vi "Sensor_Reads.vi"() -> ()   [LabVIEW 2020]
uses:
  <vilib>/Rock Robotics/WPI/ThirdParty/Phoenix-LabVIEW/Pigeon IMU/CTRE_PigeonIMU_TareType.ctl
  <vilib>/Rock Robotics/Network Tables/NT Read Number.vi
  Globals/Sensor_Values.vi
  Hardware/Drive/Drive_Hardware_Globals.vi
  Globals/Drive_Globals.vi
  <vilib>/Rock Robotics/Network Tables/NT Write Number.vi
  <vilib>/Rock Robotics/WPI/ThirdParty/Phoenix-LabVIEW/Pigeon IMU/CTRE_PigeonIMU_GetYPR.vi
  <vilib>/Rock Robotics/WPI/ThirdParty/Phoenix-LabVIEW/Motor Controller/Get/CTRE_Phoenix_MotorController_GetSelectedSensorData.vi
  <vilib>/Rock Robotics/WPI/ThirdParty/Phoenix-LabVIEW/CANCoder/Get/CTRE_Phoenix_CANcoder_GetSensorData.vi
panel:
  in  "Back_Right_Zero":i32=2431
  out "back right raw":i32=2431
  out "BR mod":i32=2431
  in  "Back_Left_Zero":i32=2431
  out "back left raw":i32=2431
  out "BL mod":i32=2431
  in  "Front_Left_Zero":i32=2431
  out "front left raw":i32=2431
  out "FL mod":i32=2431
  in  "Front_Right_Zero":i32=2431
  out "front right raw":i32=2431
  out "FR mod":i32=2431
  # "e"
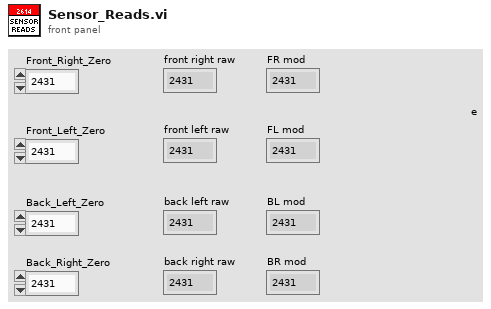
[diagram p1: front panel]
types:
  T1 = typedef "CTRE_Phoenix_CANcoder_DeviceRef.ctl" = cluster{"DeviceStatus":errorcluster, "Device Number":u8, "Handle":u64, "UsageFrame":u32, "Library Path":path}
  T2 = typedef "WPI_MotorControlDeviceRef.ctl" = cluster{"DeviceStatus":errorcluster, "Type":T3, "PWM":cluster{"PWM Channel":T4, "DeadBand":T5}, "CAN":cluster{"Device Number":u8, "SetOutput VI Ref":variant, "GetOutput VI Ref":variant, "Enable VI Ref":variant, "Disable VI Ref":variant, "Data":variant}, "Invert":bool, "DIO PWM":cluster{"PWM \"Enable\" Channel":T4, "DIOChannel":T6, "PWM Rate":dbl}}
  T3 = typedef "WPI_MotorControlType.ctl" = enum16{"PWM", "CAN", "DIO PWM"}
  T4 = typedef "FPGA_DIOPWMChannel.ctl" = enum8{"PWM 0", "PWM 1", "PWM 2", "PWM 3", "PWM 4", "PWM 5", "PWM 6", "PWM 7", "PWM 8", "PWM 9", "PWM MXP 0", "PWM MXP 1", "PWM MXP 2", "PWM MXP 3", "PWM MXP 4", "PWM MXP 5", "PWM MXP 6", "PWM MXP 7", "PWM MXP 8", "PWM MXP 9", "Invalid"}
  T5 = typedef "WPI_PWMDeadband.ctl" = cluster{"Name":string, "maxPositivePwm":i32, "minPositivePwm":i32, "centerPwm":i32, "maxNegativePwm":i32, "minNegativePwm":i32, "angularRange":u16}
  T6 = typedef "FPGA_DIOChannel.ctl" = enum8{"DIO 0", "DIO 1", "DIO 2", "DIO 3", "DIO 4", "DIO 5", "DIO 6", "DIO 7", "DIO 8", "DIO 9", "DIO MXP 0", "DIO MXP 1", "DIO MXP 2", "DIO MXP 3", "DIO MXP 4", "DIO MXP 5", "DIO MXP 6", "DIO MXP 7", "DIO MXP 8", "DIO MXP 9", "DIO MXP 10", "DIO MXP 11", "DIO MXP 12", "DIO MXP 13", "DIO MXP 14", "DIO MXP 15", "SPI Port CS1", "SPI Port CS2", "SPI Port CS3", "SPI Port MISO", "SPI Port MOSI", "Invalid"}
  T7 = typedef "CTRE_PigeonIMU_DeviceRef.ctl" = cluster{"DeviceStatus":errorcluster, "Device Number":u8, "Type":T8, "Device ID":u32, "Handle":u64, "UsageFrame":u32, "Library Path":path}
  T8 = typedef "CTRE_PigeonIMU_ConnectionType.ctl" = u32
  T9 = typedef "CTRE_PigeonIMU_TareType.ctl" = u8
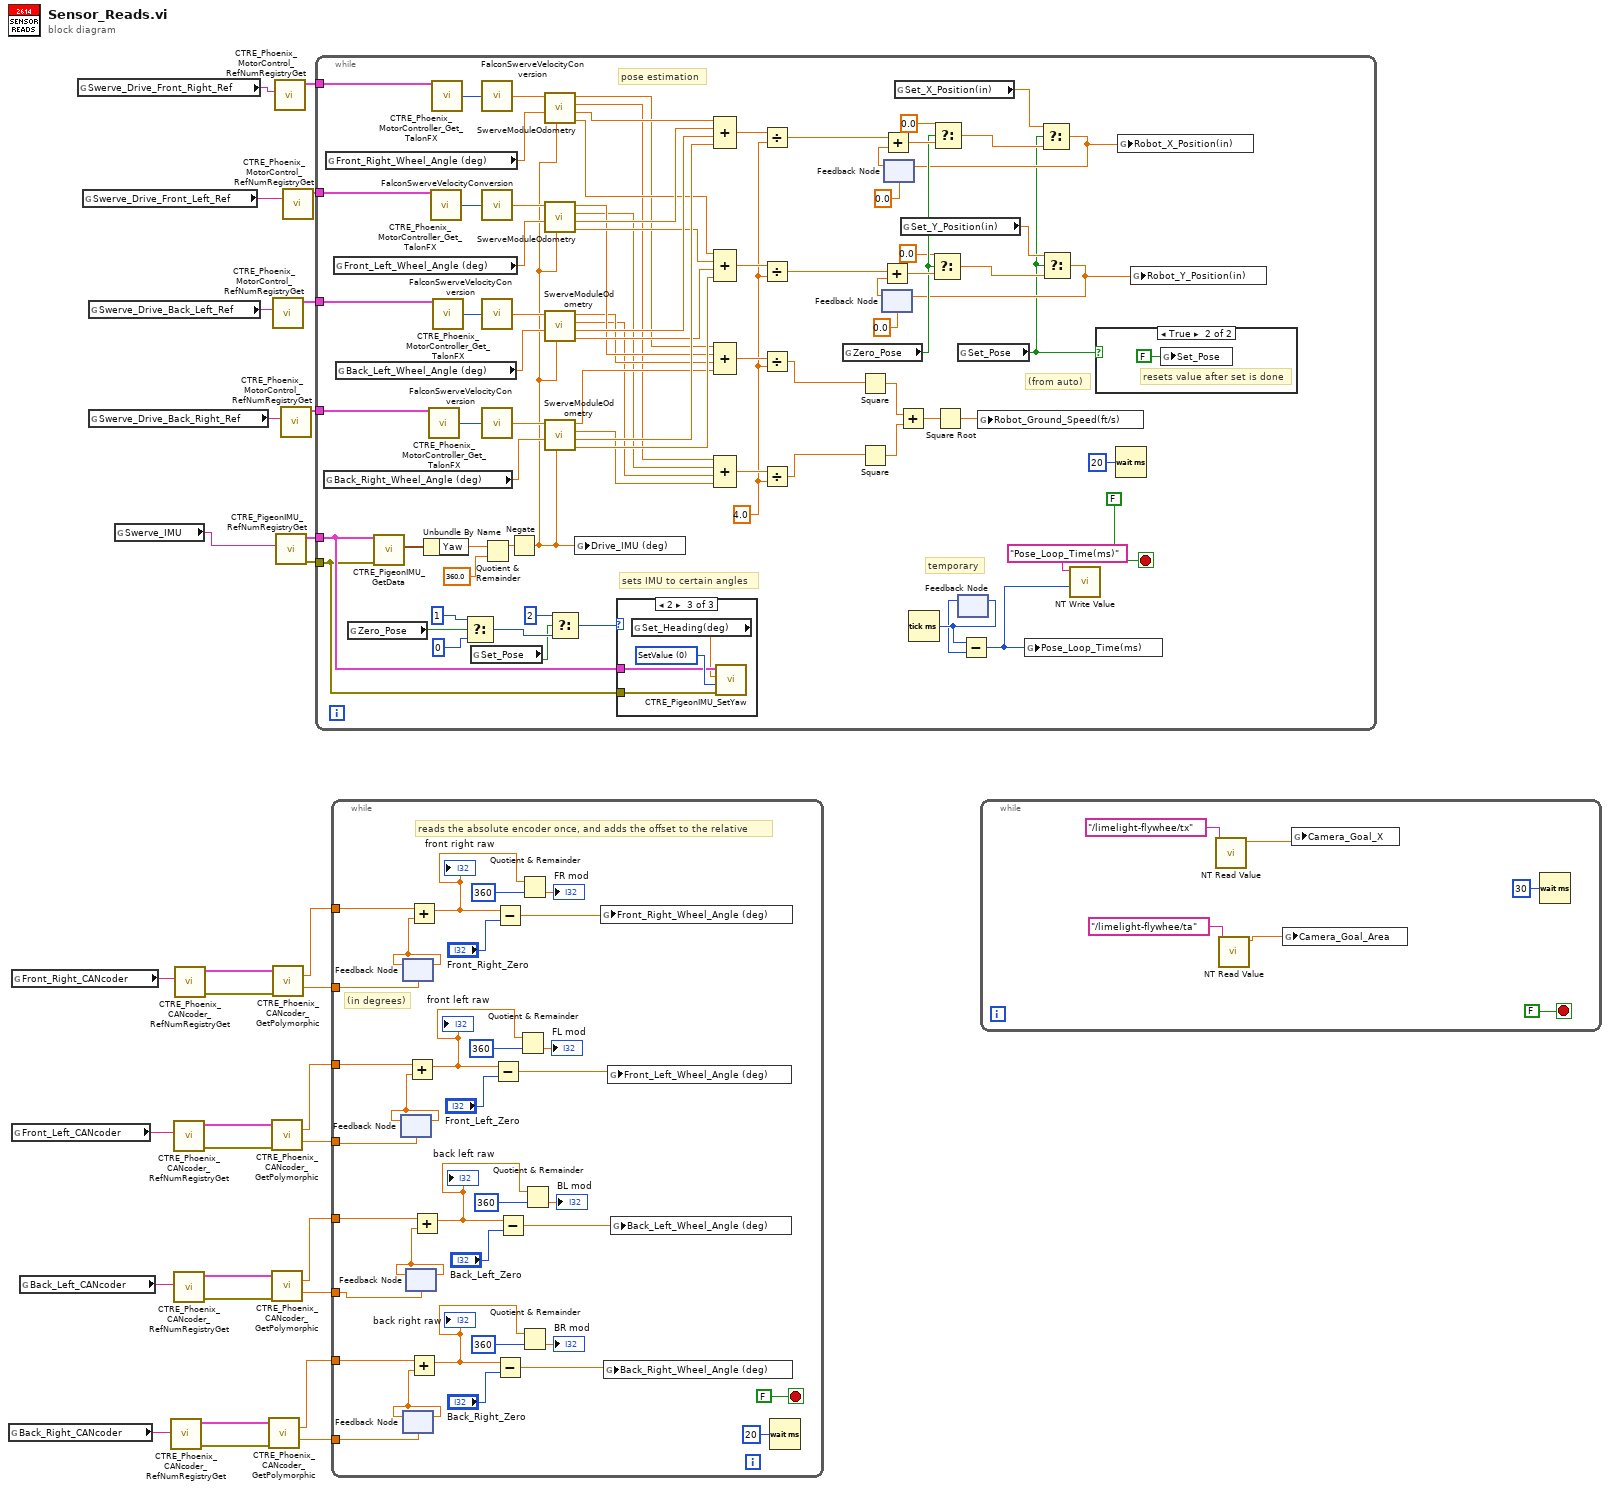
[diagram p0: block diagram]
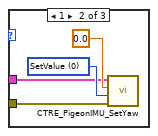
[diagram p4: hidden frame]
diagram:
  n1 = global read "Drive_Hardware_Globals.vi" "Back_Right_CANcoder"() -> (w8:string)
  n2 = global read "Drive_Hardware_Globals.vi" "Front_Right_CANcoder"() -> (w20:string)
  n3 = global read "Drive_Hardware_Globals.vi" "Front_Left_CANcoder"() -> (w10:string)
  n4 = global read "Drive_Hardware_Globals.vi" "Back_Left_CANcoder"() -> (w9:string)
  n5 = global read "Drive_Hardware_Globals.vi" "Swerve_Drive_Front_Right_Ref"() -> (w21:string)
  n6 = global read "Drive_Hardware_Globals.vi" "Swerve_Drive_Front_Left_Ref"() -> (w22:string)
  n7 = global read "Drive_Hardware_Globals.vi" "Swerve_Drive_Back_Left_Ref"() -> (w31:string)
  n8 = global read "Drive_Hardware_Globals.vi" "Swerve_Drive_Back_Right_Ref"() -> (w30:string)
  n9 = global read "Drive_Hardware_Globals.vi" "Swerve_IMU"() -> (w25:string)
  n10 = call <vilib>:"CTRE_Phoenix_CANcoder_RefNumRegistryGet.vi"("refnum name"=w8) -> ("error out"=w12:errorcluster, "CTRE_CANcoder_DeviceRef"=w11:T1)  [unwired: 9 in]
  n11 = call <vilib>:"CTRE_Phoenix_CANcoder_RefNumRegistryGet.vi"("refnum name"=w10) -> ("error out"=w16:errorcluster, "CTRE_CANcoder_DeviceRef"=w15:T1)  [unwired: 9 in]
  n12 = call <vilib>:"CTRE_Phoenix_CANcoder_RefNumRegistryGet.vi"("refnum name"=w9) -> ("error out"=w13:errorcluster, "CTRE_CANcoder_DeviceRef"=w14:T1)  [unwired: 9 in]
  n13 = call <vilib>:"CTRE_Phoenix_CANcoder_RefNumRegistryGet.vi"("refnum name"=w20) -> ("error out"=w18:errorcluster, "CTRE_CANcoder_DeviceRef"=w19:T1)  [unwired: 9 in]
  n14 = call-poly <vilib>:"CTRE_Phoenix_CANcoder_GetPolymorphic.vi"("CTRE_CANcoder_DeviceRef"=w11, "error in"=w12) -> ("Position"=w1:dbl, "Absolute Position"=w5:dbl)  [unwired: 9 in, 3 out]
  n15 = call-poly <vilib>:"CTRE_Phoenix_CANcoder_GetPolymorphic.vi"("CTRE_CANcoder_DeviceRef"=w15, "error in"=w16) -> ("Position"=w3:dbl, "Absolute Position"=w7:dbl)  [unwired: 9 in, 3 out]
  n16 = call-poly <vilib>:"CTRE_Phoenix_CANcoder_GetPolymorphic.vi"("CTRE_CANcoder_DeviceRef"=w14, "error in"=w13) -> ("Position"=w2:dbl, "Absolute Position"=w6:dbl)  [unwired: 9 in, 3 out]
  n17 = call <vilib>:"CTRE_Phoenix_MotorControl_RefNumRegistryGet.vi"("refnum name"=w31) -> ("PhoenixMotorControlDevRef"=w27:T2)  [unwired: 9 in, 1 out]
  n18 = call-poly <vilib>:"CTRE_Phoenix_CANcoder_GetPolymorphic.vi"("CTRE_CANcoder_DeviceRef"=w19, "error in"=w18) -> ("Position"=w4:dbl, "Absolute Position"=w17:dbl)  [unwired: 9 in, 3 out]
  n19 = call <vilib>:"CTRE_Phoenix_MotorControl_RefNumRegistryGet.vi"("refnum name"=w21) -> ("PhoenixMotorControlDevRef"=w29:T2)  [unwired: 9 in, 1 out]
  n20 = call <vilib>:"CTRE_PigeonIMU_RefNumRegistryGet.vi"("refnum name"=w25) -> ("error out"=w23:errorcluster, "PigeonIMUDevRef"=w24:T7)  [unwired: 9 in]
  n21 = call <vilib>:"CTRE_Phoenix_MotorControl_RefNumRegistryGet.vi"("refnum name"=w30) -> ("PhoenixMotorControlDevRef"=w26:T2)  [unwired: 9 in, 1 out]
  n22 = call <vilib>:"CTRE_Phoenix_MotorControl_RefNumRegistryGet.vi"("refnum name"=w22) -> ("PhoenixMotorControlDevRef"=w28:T2)  [unwired: 9 in, 1 out]
  n23 = while {
    tunnel: w29 -> [w112]
    tunnel: w28 -> [w111]
    tunnel: w27 -> [w110]
    tunnel: w26 -> [w109]
    tunnel: w24 -> [w54]
    tunnel: w23 -> [w53]
    stop <- FALSE stop-if-true
    w69 = 4.0 ("y")
    # "(from auto)"
    # "sets IMU to certain angles"
    # "temporary"
    # "pose estimation"
    n24 = global read "Sensor_Values.vi" "Back_Right_Wheel_Angle (deg)"() -> (w100:dbl)
    n25 = global read "Sensor_Values.vi" "Front_Right_Wheel_Angle (deg)"() -> (w56:dbl)
    n26 = global read "Sensor_Values.vi" "Front_Left_Wheel_Angle (deg)"() -> (w55:dbl)
    n27 = global read "Sensor_Values.vi" "Back_Left_Wheel_Angle (deg)"() -> (w99:dbl)
    n28 = global read "Drive_Globals.vi" "Zero_Pose"() -> (w38:bool)
    n29 = call-poly <vilib>:"CTRE_PigeonIMU_GetData.vi"("error in (no error)"=w53, "PigeonIMUDevRef"=w54) -> ("Yaw Pitch Roll"=w76:cluster{"Yaw":dbl, "Pitch":dbl, "Roll":dbl})  [unwired: 7 in, 2 out]
    n30 = Unbundle By Name(w76) -> ("Yaw"=w75:dbl)
    n31 = call-poly <vilib>:"CTRE_Phoenix_MotorController_Get_TalonFX.vi"("PhoenixMotorControlDevRef"=w109) -> ("Velocity (Raw Sensor Units per 100 ms)"=w105:i32)  [unwired: 11 in, 3 out]
    n32 = call-poly <vilib>:"CTRE_Phoenix_MotorController_Get_TalonFX.vi"("PhoenixMotorControlDevRef"=w111) -> ("Velocity (Raw Sensor Units per 100 ms)"=w107:i32)  [unwired: 11 in, 3 out]
    n33 = call-poly <vilib>:"CTRE_Phoenix_MotorController_Get_TalonFX.vi"("PhoenixMotorControlDevRef"=w112) -> ("Velocity (Raw Sensor Units per 100 ms)"=w108:i32)  [unwired: 11 in, 3 out]
    n34 = call-poly <vilib>:"CTRE_Phoenix_MotorController_Get_TalonFX.vi"("PhoenixMotorControlDevRef"=w110) -> ("Velocity (Raw Sensor Units per 100 ms)"=w106:i32)  [unwired: 11 in, 3 out]
    n35 = Select(t=1, s=w38, f=0 ("Velocity (Raw Sensor Units per 100 ms)")) -> (s? t:f=w36:i32)
    n36 = global read "Drive_Globals.vi" "Set_Pose"() -> (w34:bool)
    n37 = call "FalconSwerveVelocityConversion.vi"("Velocity (Raw Sensor Units per 100 ms)"=w108) -> ("Velocity (ft/s)"=w104:dbl)
    n38 = call "FalconSwerveVelocityConversion.vi"("Velocity (Raw Sensor Units per 100 ms)"=w107) -> ("Velocity (ft/s)"=w103:dbl)
    n39 = call "FalconSwerveVelocityConversion.vi"("Velocity (Raw Sensor Units per 100 ms)"=w106) -> ("Velocity (ft/s)"=w102:dbl)
    n40 = call "FalconSwerveVelocityConversion.vi"("Velocity (Raw Sensor Units per 100 ms)"=w105) -> ("Velocity (ft/s)"=w101:dbl)
    n41 = Quotient & Remainder(x=w75, y=360.0) -> (x-y*floor(x/y)=w57:dbl)  [unwired: 1 out]
    n42 = Negate(x=w57) -> (-x=w52:dbl)
    n43 = call "SwerveModuleOdometry.vi"("Robot Heading(deg)"=w52, "Wheel Azimuth (deg)"=w56, "Velocity (ft/s)"=w104) -> ("Delta Y (in)"=w94:dbl, "Delta X (in)"=w98:dbl, "Velocity Y (ft/s)"=w80:dbl, "Velocity X (ft/s)"=w84:dbl)  [unwired: 3 in]
    n44 = call "SwerveModuleOdometry.vi"("Robot Heading(deg)"=w52, "Wheel Azimuth (deg)"=w55, "Velocity (ft/s)"=w103) -> ("Delta Y (in)"=w93:dbl, "Delta X (in)"=w97:dbl, "Velocity Y (ft/s)"=w79:dbl, "Velocity X (ft/s)"=w83:dbl)  [unwired: 3 in]
    n45 = call "SwerveModuleOdometry.vi"("Robot Heading(deg)"=w52, "Wheel Azimuth (deg)"=w99, "Velocity (ft/s)"=w102) -> ("Delta Y (in)"=w92:dbl, "Delta X (in)"=w96:dbl, "Velocity Y (ft/s)"=w78:dbl, "Velocity X (ft/s)"=w82:dbl)  [unwired: 3 in]
    n46 = call "SwerveModuleOdometry.vi"("Robot Heading(deg)"=w52, "Wheel Azimuth (deg)"=w100, "Velocity (ft/s)"=w101) -> ("Delta Y (in)"=w91:dbl, "Delta X (in)"=w95:dbl, "Velocity Y (ft/s)"=w77:dbl, "Velocity X (ft/s)"=w81:dbl)  [unwired: 3 in]
    n47 = Select(t=2, s=w34, f=w36) -> (s? t:f=w33:i32)
    n48 = global write "Sensor_Values.vi" "Drive_IMU (deg)"(w52) -> ()
    n49 = case shown="2" w33 {
      tunnel: w54 -> [_ w115 w120]
      tunnel: w53 -> [_ w114 w119]
      frame 0, Default {
      }
      frame 1 {
        w116 = T9 0 items=["SetValue"=0, "AddOffset"=1, "MatchCompass"=2, "SetOffset"=255] ("TareType (SetValue)")
        n50 = call <vilib>:"CTRE_PigeonIMU_SetYaw.vi"("error in (no error)"=w114, "TareType (SetValue)"=w116, "Value"=0.0, "PigeonIMUDevRef"=w115) -> ()  [unwired: 6 in, 2 out]
      }
      frame 2 {
        w121 = T9 0 items=["SetValue"=0, "AddOffset"=1, "MatchCompass"=2, "SetOffset"=255] ("TareType (SetValue)")
        n51 = global read "Drive_Globals.vi" "Set_Heading(deg)"() -> (w118:dbl)
        n52 = call <vilib>:"CTRE_PigeonIMU_SetYaw.vi"("error in (no error)"=w119, "TareType (SetValue)"=w121, "Value"=w118, "PigeonIMUDevRef"=w120) -> ()  [unwired: 6 in, 2 out]
      }
    }
    n53 = Compound Arithmetic op=ADD(w98, w97, w96, w95) -> (w73:dbl)
    n54 = Compound Arithmetic op=ADD(w94, w93, w92, w91) -> (w72:dbl)
    n55 = Compound Arithmetic op=ADD(w84, w83, w82, w81) -> (w71:dbl)
    n56 = Compound Arithmetic op=ADD(w80, w79, w78, w77) -> (w70:dbl)
    n57 = Divide(x=w73, y=w69) -> (x/y=w48:dbl)
    n58 = Divide(x=w72, y=w69) -> (x/y=w68:dbl)
    n59 = Divide(x=w71, y=w69) -> (x/y=w59:dbl)
    n60 = Divide(x=w70, y=w69) -> (x/y=w58:dbl)
    n61 = global read "Drive_Globals.vi" "Zero_Pose"() -> (w49:bool)
    n62 = Square(x=w59) -> (x^2=w67:dbl)
    n63 = Square(x=w58) -> (x^2=w66:dbl)
    n64 = feedback #1(0.0) -> (w87:dbl)
    n65 = Add(x=w68, y=w87) -> (x+y=w51:dbl)
    n66 = feedback #2(0.0) -> (w88:dbl)
    n67 = Add(x=w48, y=w88) -> (x+y=w50:dbl)
    n68 = global read "Drive_Globals.vi" "Set_X_Position(in)"() -> (w41:dbl)
    n69 = Add(x=w67, y=w66) -> (x+y=w65:dbl)
    n70 = global read "Drive_Globals.vi" "Set_Y_Position(in)"() -> (w40:dbl)
    n71 = Tick Count (ms)() -> (millisecond timer value=w63:u32)
    n72 = Select(t=0.0, s=w49, f=w51) -> (s? t:f=w45:dbl)
    n73 = Select(t=0.0, s=w49, f=w50) -> (s? t:f=w44:dbl)
    n74 = Square Root(x=w65) -> (sqrt(x)=w64:dbl)
    n75 = global read "Drive_Globals.vi" "Set_Pose"() -> (w32:bool)
    n76 = feedback-in #3(w63) -> ()
    n77 = feedback #3() -> (w62:u32)  [unwired: 1 in]
    n78 = Subtract(x=w63, y=w62) -> (x-y=w61:u32)
    n79 = global write "Sensor_Values.vi" "Robot_Ground_Speed(ft/s)"(w64) -> ()
    n80 = global write "Sensor_Values.vi" "Pose_Loop_Time(ms)"(w61) -> ()
    n81 = Select(t=w41, s=w32, f=w44) -> (s? t:f=w43:dbl)
    n82 = feedback-in #2(w43) -> ()
    n83 = Select(t=w40, s=w32, f=w45) -> (s? t:f=w42:dbl)
    n84 = feedback-in #1(w42) -> ()
    n85 = call-poly <vilib>:"NT Write Value.vi"("Numeric"=w61, "Name"="Pose_Loop_Time(ms)") -> ()  [unwired: 9 in, 1 out]
    n86 = case shown="True" w32 {
      frame False {
      }
      frame True {
        # "resets value after set is done"
        n87 = global write "Drive_Globals.vi" "Set_Pose"(FALSE ("Set_Pose")) -> ()
      }
    }
    n88 = Wait (ms)(milliseconds to wait=u32 20) -> ()  [unwired: 1 out]
    n89 = global write "Sensor_Values.vi" "Robot_X_Position(in)"(w43) -> ()
    n90 = global write "Sensor_Values.vi" "Robot_Y_Position(in)"(w42) -> ()
  }
  n91 = while {
    tunnel: w17 -> [w126]
    tunnel: w7 -> [w132]
    tunnel: w6 -> [w130]
    tunnel: w5 -> [w131]
    tunnel: w4 -> [w125]
    tunnel: w3 -> [w124]
    tunnel: w2 -> [w123]
    tunnel: w1 -> [w122]
    stop <- FALSE stop-if-true
    # "reads the absolute encoder once, and adds the offset to the relative"
    # "(in degrees)"
    n92 = feedback #4(w132) -> (w143:dbl)
    n93 = feedback-in #4(w143) -> ()
    n94 = feedback #5(w126) -> (w153:dbl)
    n95 = feedback-in #5(w153) -> ()
    n96 = feedback #6(w131) -> (w133:dbl)
    n97 = feedback-in #6(w133) -> ()
    n98 = feedback #7(w130) -> (w142:dbl)
    n99 = feedback-in #7(w142) -> ()
    n100 = Add(x=w124, y=w143) -> (x+y=w145:dbl)
    "front left raw" <- w145
    n101 = Add(x=w125, y=w153) -> (x+y=w151:dbl)
    "front right raw" <- w151
    n102 = Add(x=w122, y=w133) -> (x+y=w135:dbl)
    "back right raw" <- w135
    n103 = Add(x=w123, y=w142) -> (x+y=w140:dbl)
    "back left raw" <- w140
    n104 = Subtract(x=w145, y="Front_Left_Zero") -> (x-y=w129:dbl)
    n105 = Subtract(x=w151, y="Front_Right_Zero") -> (x-y=w148:dbl)
    n106 = Subtract(x=w135, y="Back_Right_Zero") -> (x-y=w127:dbl)
    n107 = Subtract(x=w140, y="Back_Left_Zero") -> (x-y=w128:dbl)
    n108 = Quotient & Remainder(x=w145, y=360 ("x+y")) -> (x-y*floor(x/y)=→"FL mod":dbl)  [unwired: 1 out]
    n109 = Quotient & Remainder(x=w151, y=360 ("x+y")) -> (x-y*floor(x/y)=→"FR mod":dbl)  [unwired: 1 out]
    n110 = Quotient & Remainder(x=w135, y=360 ("x+y")) -> (x-y*floor(x/y)=→"BR mod":dbl)  [unwired: 1 out]
    n111 = Quotient & Remainder(x=w140, y=360 ("x+y")) -> (x-y*floor(x/y)=→"BL mod":dbl)  [unwired: 1 out]
    n112 = global write "Sensor_Values.vi" "Front_Right_Wheel_Angle (deg)"(w148) -> ()
    n113 = global write "Sensor_Values.vi" "Back_Right_Wheel_Angle (deg)"(w127) -> ()
    n114 = global write "Sensor_Values.vi" "Front_Left_Wheel_Angle (deg)"(w129) -> ()
    n115 = global write "Sensor_Values.vi" "Back_Left_Wheel_Angle (deg)"(w128) -> ()
    n116 = Wait (ms)(milliseconds to wait=u32 20) -> ()  [unwired: 1 out]
  }
  n117 = while {
    stop <- FALSE stop-if-true
    n118 = call-poly <vilib>:"NT Read Value.vi"("Name"="/limelight-flywhee/tx") -> ("Numeric"=w161:dbl)  [unwired: 9 in, 1 out]
    n119 = call-poly <vilib>:"NT Read Value.vi"("Name"="/limelight-flywhee/ta") -> ("Numeric"=w160:dbl)  [unwired: 9 in, 1 out]
    n120 = global write "Sensor_Values.vi" "Camera_Goal_Area"(w160) -> ()
    n121 = global write "Sensor_Values.vi" "Camera_Goal_X"(w161) -> ()
    n122 = Wait (ms)(milliseconds to wait=u32 30) -> ()  [unwired: 1 out]
  }
